vi "SDCP - Encode Standard Message Frame Parameter.vi"(3 "error in (no error)":errorcluster, 4 "Value in":string, 5 "SMF descriptor in":T1) -> (0 "error out":errorcluster, 2 "Encoded message frame":u8[](array[numeric]))   [LabVIEW 2020]
uses:
  Typedefs/SDCP - SMF parameter descriptors.ctl
  Typedefs/SDCP - Standard Message Frames FGV - Commands.ctl
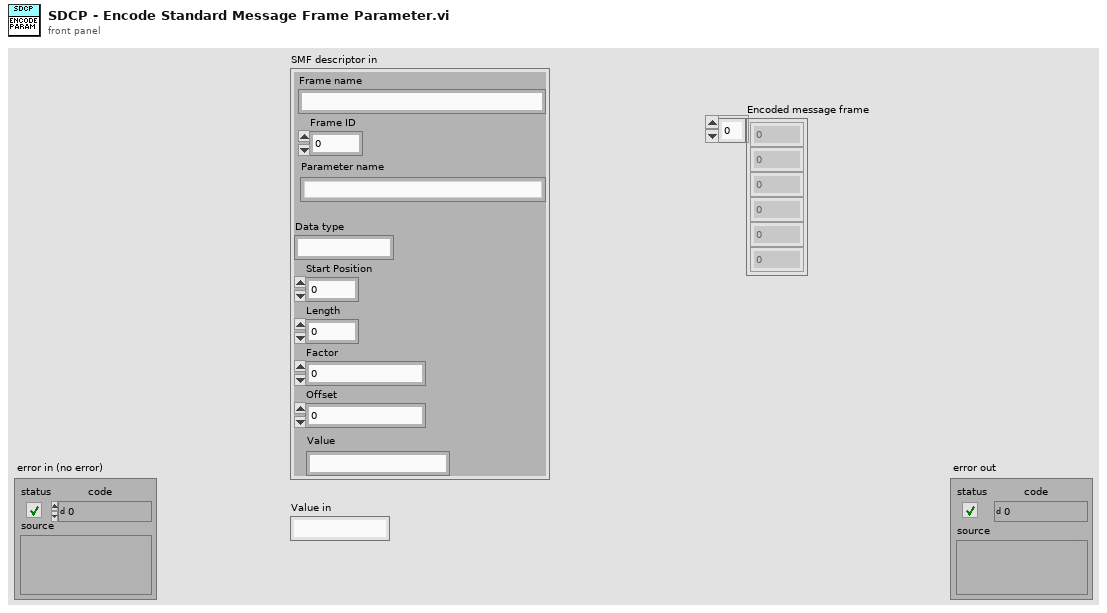
[diagram p1: front panel]
types:
  T1 = typedef "SDCP - SMF parameter descriptors.ctl" = cluster{"Frame name":string, "Frame ID":i32, "Data type":string, "Start Position":i32, "Length":i32, "Factor":dbl, "Offset":dbl, "Parameter name":string, "Value":string}
  T2 = typedef "SDCP - Standard Message Frames FGV - Commands.ctl" = enum16{"Reset", "Read", "Write", "Set Priority"}
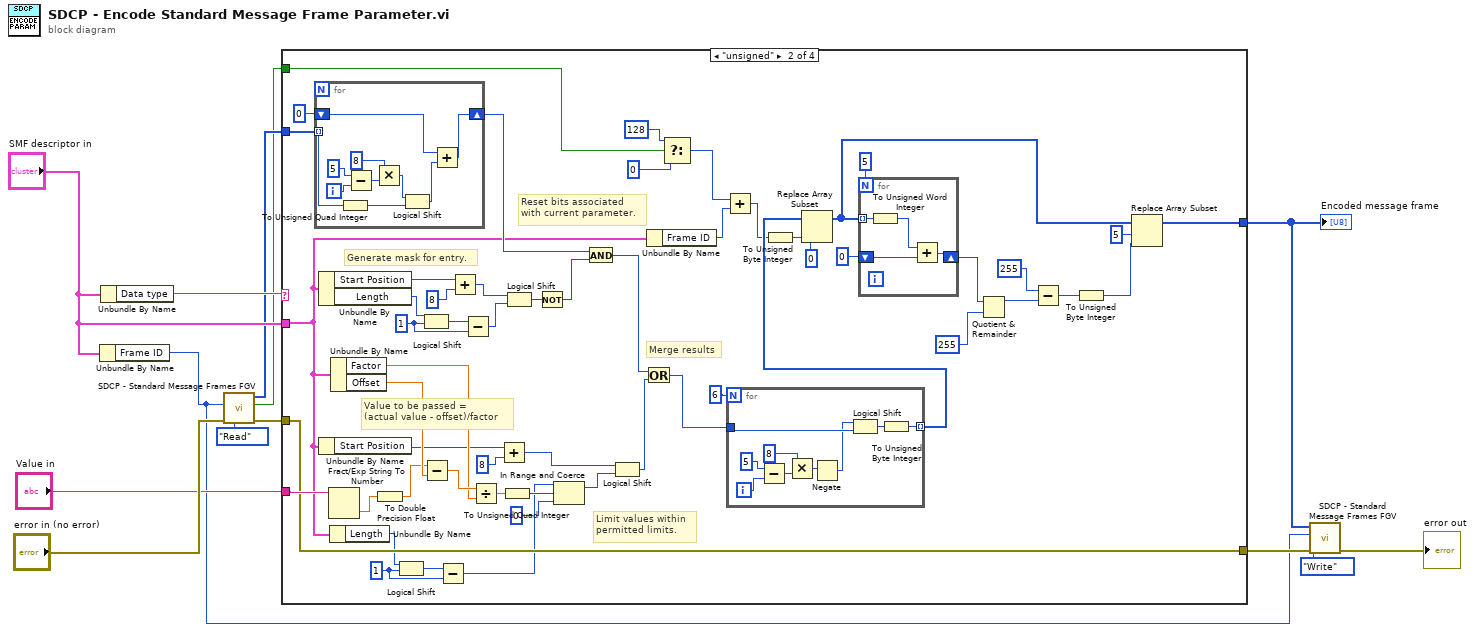
[diagram p0: block diagram]
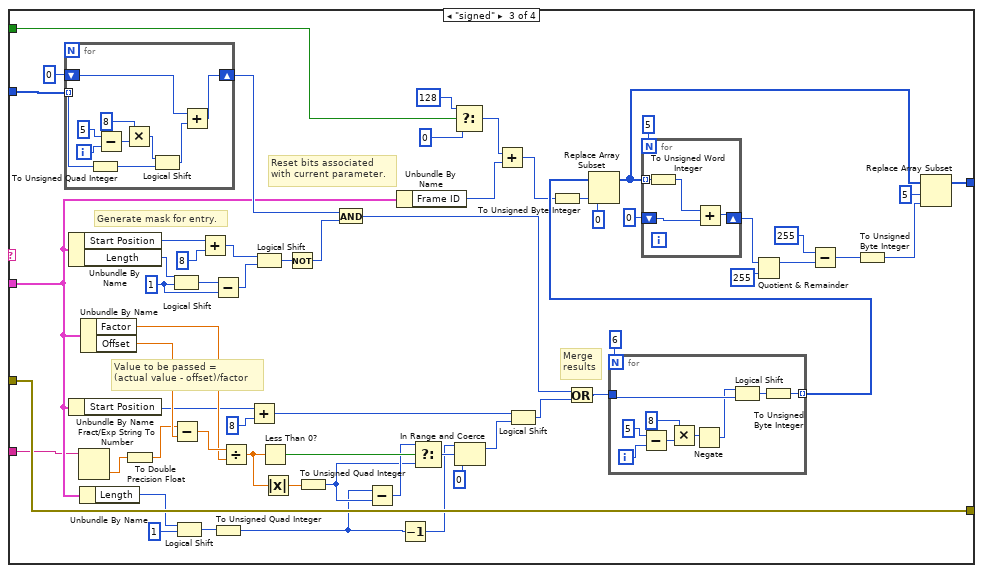
[diagram p3: hidden frame]
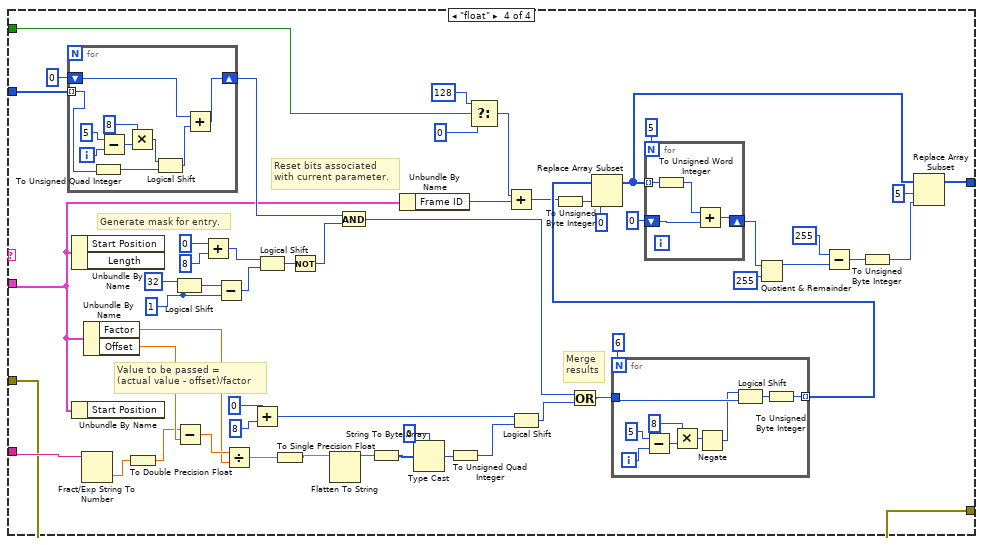
[diagram p4: hidden frame]
diagram:
  n1 = Unbundle By Name("SMF descriptor in") -> ("Frame ID"=w5:i32)
  n2 = Unbundle By Name("SMF descriptor in") -> ("Data type"=w11:string)
  n3 = call "SDCP - Standard Message Frames FGV.vi"("error in (no error)"="error in (no error)", "Command"=SDCP_-_Standard_Message_Frames_FGV_-_Commands."Read", "FID"=w5) -> ("error out"=w12:errorcluster, "Frame priority out"=w1:bool, "SMF out"=w8:u8[])  [unwired: 3 in]
  n4 = case shown="\"unsigned\"" w11 {
    tunnel: w12 -> [w15 w36 w153 w199]
    tunnel: [w15 w36 w153 w199] -> w7
    tunnel: "SMF descriptor in" -> [_ w34 w118 w201]
    tunnel: "Value in" -> [_ w70 w117 w200]
    tunnel: w8 -> [w14 w42 w119 w187]
    tunnel: [w14 w46 w116 w198] -> w6
    tunnel: w1 -> [_ w21 w101 w184]
    frame Default {
    }
    frame "unsigned" {
      w32 = u64 1
      w61 = u64 1
      # "Limit values within\npermitted limits."
      # "Merge results"
      # "Value to be passed = \n(actual value - offset)/factor"
      # "Reset bits associated\nwith current parameter."
      # "Generate mask for entry."
      n5 = for {
        tunnel: w42 -> [w86] mode=indexing
        shift-right: [w88] -> w40
        shift-left: u64 0 -> [w89]
        i -> [w85]
        n6 = To Unsigned Quad Integer(1:w86) -> (0:w87:u64)
        n7 = Subtract(x=5, y=w85) -> (x-y=w82:i32)
        n8 = Multiply(x=8, y=w82) -> (x*y=w81:i32)
        n9 = Logical Shift(y=w81, x=w87) -> (x << y=w83:u64)
        n10 = Add(x=w89, y=w83) -> (x+y=w88:u64)
      }
      n11 = Unbundle By Name(w34) -> ("Start Position"=w57:i32, "Length"=w60:i32)
      n12 = Unbundle By Name(w34) -> ("Start Position"=w65:i32)
      n13 = Fract/Exp String To Number(string=w70) -> (number=w45:dbl)  [unwired: 3 in, 1 out]
      n14 = Unbundle By Name(w34) -> ("Length"=w31:i32)
      n15 = Unbundle By Name(w34) -> ("Factor"=w66:dbl, "Offset"=w69:dbl)
      n16 = To Double Precision Float(number=w45) -> (double precision float=w68:dbl)
      n17 = Logical Shift(y=w31, x=w32) -> (x << y=w33:u64)
      n18 = Logical Shift(y=w60, x=w61) -> (x << y=w62:u64)
      n19 = Subtract(x=w68, y=w69) -> (x-y=w67:dbl)
      n20 = Subtract(x=w33, y=w32) -> (x-y=w28:u64)
      n21 = Add(x=w57, y=8) -> (x+y=w44:i32)
      n22 = Subtract(x=w62, y=w61) -> (x-y=w35:u64)
      n23 = Divide(x=w67, y=w66) -> (x/y=w30:dbl)
      n24 = Add(x=w65, y=8) -> (x+y=w63:i32)
      n25 = To Unsigned Quad Integer(1:w30) -> (0:w29:u64)
      n26 = Logical Shift(y=w44, x=w35) -> (x << y=w59:u64)
      n27 = Not(x=w59) -> (.not. x?=w58:u64)
      n28 = In Range and Coerce(upper limit=w28, x=w29, lower limit=u64 0) -> (coerced(x)=w26:u64)  [unwired: 1 out]
      n29 = And(x=w40, y=w58) -> (x .and. y?=w56:u64)
      n30 = Logical Shift(y=w63, x=w26) -> (x << y=w55:u64)
      n31 = Or(x=w56, y=w55) -> (x .or. y?=w39:u64)
      n32 = Unbundle By Name(w34) -> ("Frame ID"=w25:i32)
      n33 = Select(t=128, s=w21, f=0) -> (s? t:f=w20:i32)
      n34 = Add(x=w20, y=w25) -> (x+y=w24:i32)
      n35 = for {
        N: 6 -> [_]
        tunnel: w39 -> [w75]
        tunnel: [w71] -> w37 mode=indexing
        i -> [w76]
        n36 = Subtract(x=5, y=w76) -> (x-y=w78:i32)
        n37 = Multiply(x=8, y=w78) -> (x*y=w74:i32)
        n38 = Negate(x=w74) -> (-x=w73:i32)
        n39 = Logical Shift(y=w73, x=w75) -> (x << y=w72:u64)
        n40 = To Unsigned Byte Integer(number=w72) -> (unsigned 8bit integer=w71:u8)
      }
      n41 = To Unsigned Byte Integer(number=w24) -> (unsigned 8bit integer=w49:u8)
      n42 = Replace Array Subset(array=w37, new element=w49, index=0) -> (w48:u8[])
      n43 = for {
        N: 5 -> [_]
        tunnel: w48 -> [w92] mode=indexing
        shift-right: [w91] -> w52
        shift-left: u16 0 -> [w93]
        n44 = To Unsigned Word Integer(number=w92) -> (unsigned 16bit integer=w90:u16)
        n45 = Add(x=w90, y=w93) -> (x+y=w91:u16)
      }
      n46 = Quotient & Remainder(x=w52, y=u16 255) -> (x-y*floor(x/y)=w19:u16)  [unwired: 1 out]
      n47 = Subtract(x=u16 255, y=w19) -> (x-y=w17:u16)
      n48 = To Unsigned Byte Integer(number=w17) -> (unsigned 8bit integer=w16:u8)
      n49 = Replace Array Subset(array=w48, new element=w16, index=5) -> (w46:u8[])
    }
    frame "signed" {
      w144 = u64 1
      # "Merge \nresults"
      # "Value to be passed = \n(actual value - offset)/factor"
      # "Reset bits associated\nwith current parameter."
      # "Generate mask for entry."
      n50 = for {
        tunnel: w119 -> [w169] mode=indexing
        shift-right: [w171] -> w125
        shift-left: u64 0 -> [w172]
        i -> [w168]
        n51 = To Unsigned Quad Integer(1:w169) -> (0:w170:u64)
        n52 = Subtract(x=5, y=w168) -> (x-y=w165:i32)
        n53 = Multiply(x=8, y=w165) -> (x*y=w164:i32)
        n54 = Logical Shift(y=w164, x=w170) -> (x << y=w166:u64)
        n55 = Add(x=w172, y=w166) -> (x+y=w171:u64)
      }
      n56 = Unbundle By Name(w118) -> ("Start Position"=w140:i32, "Length"=w143:i32)
      n57 = Unbundle By Name(w118) -> ("Start Position"=w148:i32)
      n58 = Fract/Exp String To Number(string=w117) -> (number=w129:dbl)  [unwired: 3 in, 1 out]
      n59 = Unbundle By Name(w118) -> ("Length"=w115:i32)
      n60 = Unbundle By Name(w118) -> ("Factor"=w149:dbl, "Offset"=w152:dbl)
      n61 = To Double Precision Float(number=w129) -> (double precision float=w151:dbl)
      n62 = Logical Shift(y=w143, x=w144) -> (x << y=w145:u64)
      n63 = Subtract(x=w151, y=w152) -> (x-y=w150:dbl)
      n64 = Logical Shift(y=w115, x=u64 1) -> (x << y=w112:u64)
      n65 = Add(x=w140, y=8) -> (x+y=w128:i32)
      n66 = Subtract(x=w145, y=w144) -> (x-y=w121:u64)
      n67 = To Unsigned Quad Integer(1:w112) -> (0:w107:u64)
      n68 = Divide(x=w150, y=w149) -> (x/y=w114:dbl)
      n69 = Add(x=w148, y=8) -> (x+y=w146:i32)
      n70 = Logical Shift(y=w128, x=w121) -> (x << y=w142:u64)
      n71 = Less Than 0?(x=w114) -> (x < 0?=w111:bool)
      n72 = Absolute Value(x=w114) -> (abs(x)=w113:dbl)
      n73 = Not(x=w142) -> (.not. x?=w141:u64)
      n74 = To Unsigned Quad Integer(1:w113) -> (0:w109:u64)
      n75 = And(x=w125, y=w141) -> (x .and. y?=w139:u64)
      n76 = Subtract(x=w107, y=w109) -> (x-y=w110:u64)
      n77 = Unbundle By Name(w118) -> ("Frame ID"=w99:i32)
      n78 = Decrement(x=w107) -> (x-1=w106:u64)
      n79 = Select(t=w110, s=w111, f=w109) -> (s? t:f=w108:u64)
      n80 = Select(t=128, s=w101, f=0) -> (s? t:f=w100:i32)
      n81 = In Range and Coerce(upper limit=w106, x=w108, lower limit=u64 0) -> (coerced(x)=w104:u64)  [unwired: 1 out]
      n82 = Add(x=w100, y=w99) -> (x+y=w98:i32)
      n83 = Logical Shift(y=w146, x=w104) -> (x << y=w138:u64)
      n84 = To Unsigned Byte Integer(number=w98) -> (unsigned 8bit integer=w132:u8)
      n85 = Or(x=w139, y=w138) -> (x .or. y?=w124:u64)
      n86 = for {
        N: 6 -> [_]
        tunnel: w124 -> [w158]
        tunnel: [w154] -> w122 mode=indexing
        i -> [w159]
        n87 = Subtract(x=5, y=w159) -> (x-y=w161:i32)
        n88 = Multiply(x=8, y=w161) -> (x*y=w157:i32)
        n89 = Negate(x=w157) -> (-x=w156:i32)
        n90 = Logical Shift(y=w156, x=w158) -> (x << y=w155:u64)
        n91 = To Unsigned Byte Integer(number=w155) -> (unsigned 8bit integer=w154:u8)
      }
      n92 = Replace Array Subset(array=w122, new element=w132, index=0) -> (w131:u8[])
      n93 = for {
        N: 5 -> [_]
        tunnel: w131 -> [w175] mode=indexing
        shift-right: [w174] -> w135
        shift-left: u16 0 -> [w176]
        n94 = To Unsigned Word Integer(number=w175) -> (unsigned 16bit integer=w173:u16)
        n95 = Add(x=w173, y=w176) -> (x+y=w174:u16)
      }
      n96 = Quotient & Remainder(x=w135, y=u16 255) -> (x-y*floor(x/y)=w97:u16)  [unwired: 1 out]
      n97 = Subtract(x=u16 255, y=w97) -> (x-y=w96:u16)
      n98 = To Unsigned Byte Integer(number=w96) -> (unsigned 8bit integer=w94:u8)
      n99 = Replace Array Subset(array=w131, new element=w94, index=5) -> (w116:u8[])
    }
    frame "float" {
      w223 = u64 1
      # "Merge \nresults"
      # "Value to be passed = \n(actual value - offset)/factor"
      # "Reset bits associated\nwith current parameter."
      # "Generate mask for entry."
      n100 = for {
        shift-right: [w248] -> w206
        shift-left: u64 0 -> [w249]
        tunnel: w187 -> [w240] mode=indexing
        i -> [w246]
        n101 = To Unsigned Quad Integer(1:w240) -> (0:w247:u64)
        n102 = Subtract(x=5, y=w246) -> (x-y=w243:i32)
        n103 = Multiply(x=8, y=w243) -> (x*y=w242:i32)
        n104 = Logical Shift(y=w242, x=w247) -> (x << y=w244:u64)
        n105 = Add(x=w249, y=w244) -> (x+y=w248:u64)
      }
      n106 = Unbundle By Name(w201) -> ()  [unwired: 2 out]
      n107 = Unbundle By Name(w201) -> ()  [unwired: 1 out]
      n108 = Fract/Exp String To Number(string=w200) -> (number=w210:dbl)  [unwired: 3 in, 1 out]
      n109 = Unbundle By Name(w201) -> ("Factor"=w227:dbl, "Offset"=w230:dbl)
      n110 = To Double Precision Float(number=w210) -> (double precision float=w229:dbl)
      n111 = Logical Shift(y=i16 32, x=w223) -> (x << y=w224:u64)
      n112 = Subtract(x=w229, y=w230) -> (x-y=w228:dbl)
      n113 = Add(x=0, y=8) -> (x+y=w209:i32)
      n114 = Subtract(x=w224, y=w223) -> (x-y=w202:u64)
      n115 = Divide(x=w228, y=w227) -> (x/y=w197:dbl)
      n116 = Add(x=0, y=8) -> (x+y=w225:i32)
      n117 = Logical Shift(y=w209, x=w202) -> (x << y=w222:u64)
      n118 = To Single Precision Float(number=w197) -> (single precision float=w196:sgl)
      n119 = Not(x=w222) -> (.not. x?=w221:u64)
      n120 = Flatten To String(anything=w196) -> (data string=w195:string)  [unwired: 3 in, 2 out]
      n121 = And(x=w206, y=w221) -> (x .and. y?=w220:u64)
      n122 = String To Byte Array(string=w195) -> (unsigned byte array=w194:u8[])
      n123 = Unbundle By Name(w201) -> ("Frame ID"=w183:i32)
      n124 = Type Cast(type=u32 0, x=w194) -> (*(type *) &x=w189:u32)
      n125 = To Unsigned Quad Integer(1:w189) -> (0:w188:u64)
      n126 = Select(t=128, s=w184, f=0) -> (s? t:f=w182:i32)
      n127 = Add(x=w182, y=w183) -> (x+y=w181:i32)
      n128 = Logical Shift(y=w225, x=w188) -> (x << y=w219:u64)
      n129 = To Unsigned Byte Integer(number=w181) -> (unsigned 8bit integer=w213:u8)
      n130 = Or(x=w220, y=w219) -> (x .or. y?=w205:u64)
      n131 = for {
        N: 6 -> [_]
        tunnel: w205 -> [w235]
        tunnel: [w231] -> w203 mode=indexing
        i -> [w236]
        n132 = Subtract(x=5, y=w236) -> (x-y=w238:i32)
        n133 = Multiply(x=8, y=w238) -> (x*y=w234:i32)
        n134 = Negate(x=w234) -> (-x=w233:i32)
        n135 = Logical Shift(y=w233, x=w235) -> (x << y=w232:u64)
        n136 = To Unsigned Byte Integer(number=w232) -> (unsigned 8bit integer=w231:u8)
      }
      n137 = Replace Array Subset(array=w203, new element=w213, index=0) -> (w212:u8[])
      n138 = for {
        N: 5 -> [_]
        tunnel: w212 -> [w251] mode=indexing
        shift-right: [w252] -> w216
        shift-left: u16 0 -> [w253]
        n139 = To Unsigned Word Integer(number=w251) -> (unsigned 16bit integer=w250:u16)
        n140 = Add(x=w250, y=w253) -> (x+y=w252:u16)
      }
      n141 = Quotient & Remainder(x=w216, y=u16 255) -> (x-y*floor(x/y)=w180:u16)  [unwired: 1 out]
      n142 = Subtract(x=u16 255, y=w180) -> (x-y=w178:u16)
      n143 = To Unsigned Byte Integer(number=w178) -> (unsigned 8bit integer=w177:u8)
      n144 = Replace Array Subset(array=w212, new element=w177, index=5) -> (w198:u8[])
    }
  }
  "Encoded message frame" <- w6
  n145 = call "SDCP - Standard Message Frames FGV.vi"("error in (no error)"=w7, "Command"=SDCP_-_Standard_Message_Frames_FGV_-_Commands."Write", "FID"=w5, "SMF in"=w6) -> ("error out"=→"error out":errorcluster)  [unwired: 2 in, 2 out]
